vi "Data Publishing Service Launcher.vi"(10 "NIVS.Workspace Event":refnum<event-registration>, 11 "NIVS.Gateway IP Address":string="localhost") -> (0 "error out":errorcluster)   [LabVIEW 2024, in "Data Publishing Service Launcher.lvlib"]
uses:
  Data Publishing Service Support.llb/Data Publishing Service Launcher.lvlib
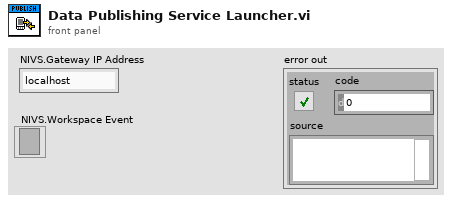
[diagram p1: front panel]
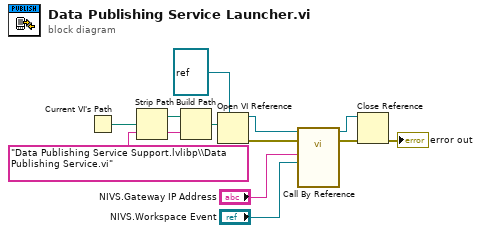
[diagram p0: block diagram]
diagram:
  n1 = Current VI's Path() -> (path=w11:path)
  n2 = Strip Path(path=w11) -> (stripped path=w10:path)  [unwired: 1 out]
  n3 = Build Path(base path=w10, name or relative path="Data Publishing Service Support.lvlibp\\Data Publishing Service.vi") -> (appended path=w1:path)
  n4 = Open VI Reference(type specifier VI Refnum (for type only)=refnum<vi> refnum, vi path=w1) -> (vi reference=w8:refnum<vi>, error out=w7:errorcluster)  [unwired: 4 in]
  n5 = call-by-ref "?"(reference=w8, error in=w7, "NIVS.Workspace Event"="NIVS.Workspace Event", "NIVS.Gateway IP Address"="NIVS.Gateway IP Address") -> (reference out=w5:refnum<vi>, error out=w6:errorcluster)  [unwired: 10 in]
  n6 = Close Reference(reference=w5, error in (no error)=w6) -> (error out=→"error out":errorcluster)
